vi "Destroy Local Events.vi"(8 "error in":errorcluster, 11 "Local Events":T1) -> (0 "error out":errorcluster)   [LabVIEW 2020, in "Monochromator.lvlib" / "Local Events.lvlib"]
doc: "____\nPantherLAB Templates 1.0.0.5\nCopyright (c) 2022, PantherLAB"
uses:
  Local Events.lvlib
  Local Events--cluster.ctl
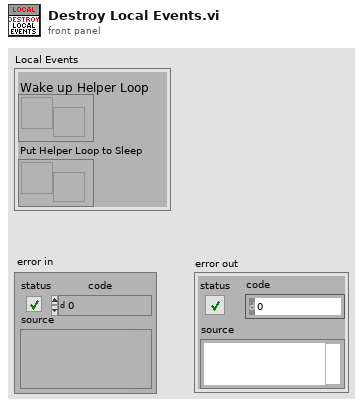
[diagram p1: front panel]
types:
  T1 = typedef "Monochromator.lvlib/Local Events.lvlib/Local Events--cluster.ctl" = cluster{"Wake up Helper Loop":refnum<user-event>, "Put Helper Loop to Sleep":refnum<user-event>}
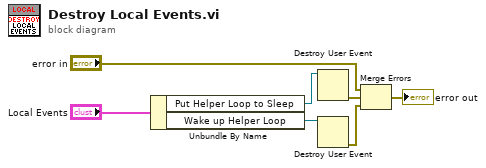
[diagram p0: block diagram]
diagram:
  n1 = Unbundle By Name("Local Events") -> ("Put Helper Loop to Sleep"=w1:refnum<user-event>, "Wake up Helper Loop"=w2:refnum<user-event>)
  n2 = Destroy User Event(user event=w1) -> (error out=w6:errorcluster)  [unwired: 1 in]
  n3 = Destroy User Event(user event=w2) -> (error out=w5:errorcluster)  [unwired: 1 in]
  n4 = Merge Errors("error in", w6, w5) -> (→"error out":errorcluster)
